vi "_Open VI Reference Without Loading Deps.vi"(8 "error in (no error)":errorcluster, 9 "Options":i32=2 format="%.0x", 10 "CSM-VI":path) -> (0 "error out":errorcluster, 3 "VI Out":refnum<vi>)   [LabVIEW 2017, in "CSM-Helper API with lvcsm Support.lvlib"]
uses:
  CSM-Helper API with lvcsm Support.lvlib
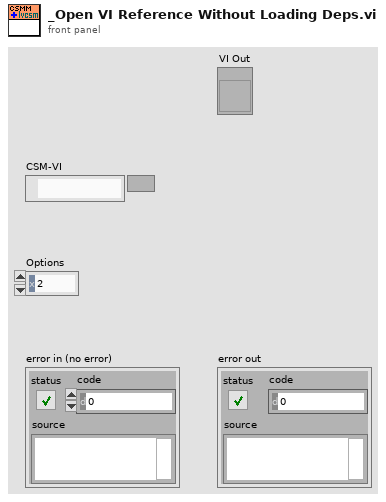
[diagram p1: front panel]
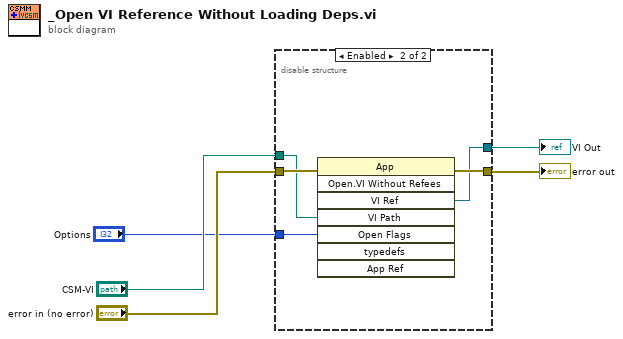
[diagram p0: block diagram]
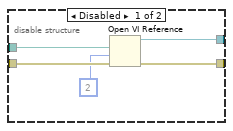
[diagram p2: hidden frame]
diagram:
  n1 = disable-structure "Diagram Disable Structure" shown="Enabled" {
    disable-tunnel: "error in (no error)" -> [w10 w15]
    disable-tunnel: [w9 w14] -> w3
    disable-tunnel: "CSM-VI" -> [w8 w13]
    disable-tunnel: [w6 w12] -> w5
    disable-tunnel: "Options" -> [_ w11]
    frame Disabled {
      n2 = Open VI Reference(vi path=w8, options=2, error in (no error)=w10) -> (vi reference=w6:refnum<vi>, error out=w9:errorcluster)  [unwired: 3 in]
    }
    frame Enabled {
      n3 = invoke class="App" method="Open.VI Without Refees"(error in=w15, "VI Path"=w13, "Open Flags"=w11) -> (error out=w14:errorcluster, "VI Ref"=w12:refnum<vi>)  [unwired: 5 in, 6 out]
    }
  }
  "VI Out" <- w5
  "error out" <- w3
